vi "Begins with Qualified Name.vi"(9 "beginning name":string, 11 "name":string) -> (1 "ending name":string, 3 "begins with name":bool)   [LabVIEW 2021, in "MeasurementService Editor.lvlib"]
uses:
  MeasurementService Editor.lvlib
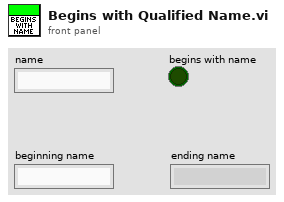
[diagram p1: front panel]
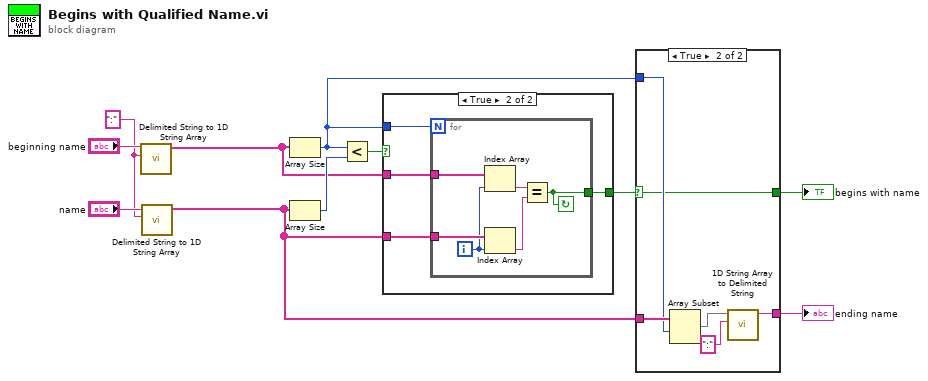
[diagram p0: block diagram]
diagram:
  w4 = ":" ("format string")
  n1 = call <vilib>:"Delimited String to 1D String Array.vi"("delimiter"=w4, "delimited string"="beginning name") -> ("string array"=w3:string[])  [unwired: 9 in]
  n2 = call <vilib>:"Delimited String to 1D String Array.vi"("delimiter"=w4, "delimited string"="name") -> ("string array"=w2:string[])  [unwired: 9 in]
  n3 = Array Size(array=w3) -> (size(s)=w8:i32)
  n4 = Array Size(array=w2) -> (size(s)=w11:i32)
  n5 = Less?(x=w8, y=w11) -> (x < y?=w10:bool)
  n6 = case shown="True" w10 {
    selector: w10 -> [w12 _]
    tunnel: w2 -> [_ w15]
    tunnel: w3 -> [_ w16]
    tunnel: [w12 w14] -> w9
    tunnel: w8 -> [_ w13]
    frame False {
    }
    frame True {
      n7 = for {
        N: w13 -> [_]
        tunnel: w16 -> [w22]
        tunnel: w15 -> [w18]
        tunnel: [w21] -> w14
        i -> [w17]
        stop <- w21 continue-if-true
        n8 = Index Array(array=w22, index=w17) -> (element=w20:string)
        n9 = Index Array(array=w18, index=w17) -> (element=w19:string)
        n10 = Equal?(x=w20, y=w19) -> (x = y?=w21:bool)
      }
    }
  }
  n11 = case shown="True" w9 {
    selector: w9 -> [w23 w27]
    tunnel: [w23 w27] -> w7
    tunnel: w2 -> [_ w29]
    tunnel: w8 -> [_ w28]
    tunnel: [_ w24] -> w1
    frame False {
    }
    frame True {
      n12 = Array Subset(array=w29, index=w28) -> (w26:string[])  [unwired: 1 in]
      n13 = call <vilib>:"1D String Array to Delimited String.vi"("delimiter"=":", "string array"=w26) -> ("delimited string"=w24:string)  [unwired: 9 in]
    }
  }
  "ending name" <- w1
  "begins with name" <- w7
